vi "UpdateSqueezeRelease.vi"(6 "valley":bool, 7 "valley 2":bool, 9 "peak":bool, 10 "peak 2":bool, 11 "Loop Data":T1) -> (3 "DataLoop":T1)   [LabVIEW 2016]
doc: "updates the number of squeezes nad releases since start of session"
uses:
  DataLoopCluster.ctl
  SignalType.ctl
  range_cluster.ctl
  <userlib>/_OpenG.lib/array/array.llb/Filter 1D Array with Scalar (String)__ogtk.vi
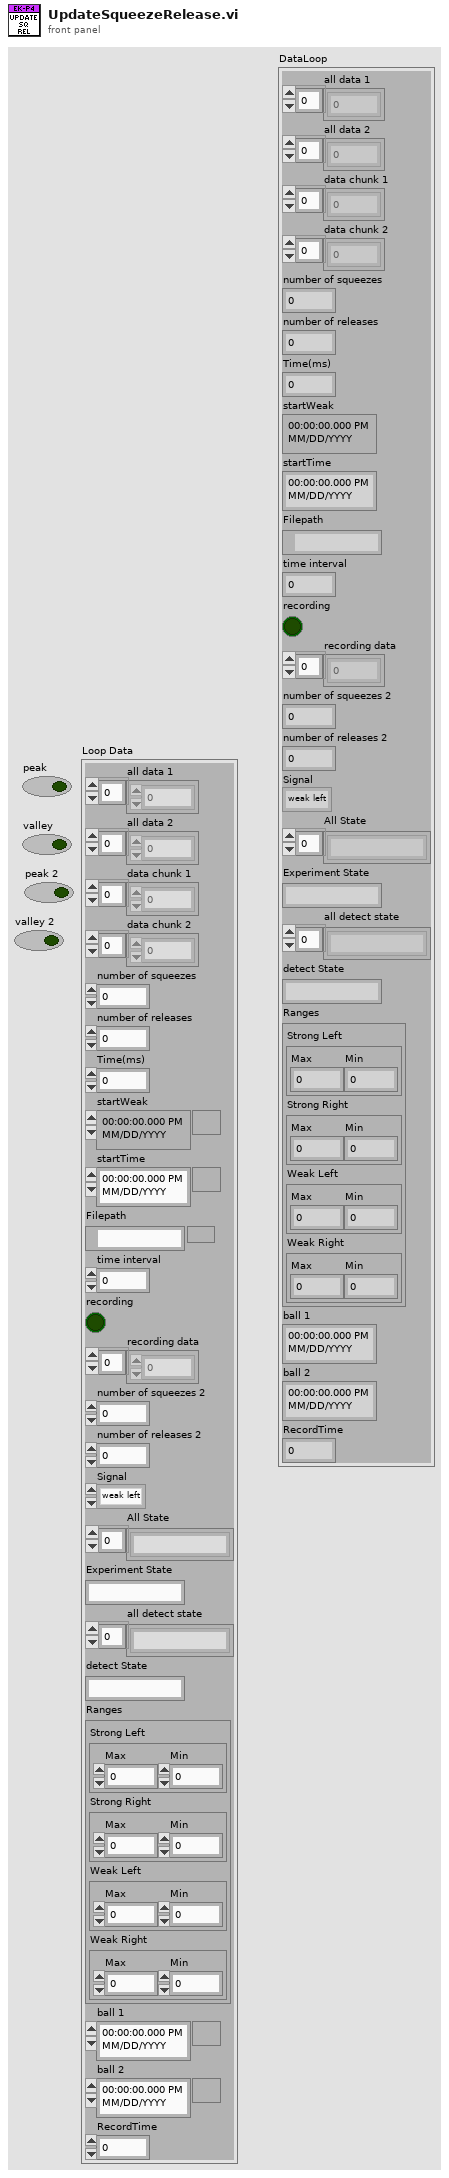
[diagram p1: front panel]
types:
  T1 = typedef "DataLoopCluster.ctl" = cluster{"all data 1":dbl[], "all data 2":dbl[], "data chunk 1":dbl[], "data chunk 2":dbl[], "number of squeezes":u16, "number of releases":u16, "Time(ms)":i64, "startWeak":timestamp, "startTime":timestamp, "Filepath":path, "time interval":u16, "recording":bool, "recording data":dbl[], "number of squeezes 2":u16, "number of releases 2":u16, "Signal":T2, "All State":string[], "Experiment State":string, "all detect state":string[], "detect State":string, "Ranges":cluster{"Strong Left":T3, "Strong Right":T3, "Weak Left":T3, "Weak Right":T3}, "ball 1":timestamp, "ball 2":timestamp, "RecordTime":u16}
  T2 = typedef "SignalType.ctl" = enum16{"weak left", "weak right", "strong left", "strong right"}
  T3 = typedef "range_cluster.ctl" = cluster{"Max":dbl, "Min":dbl}
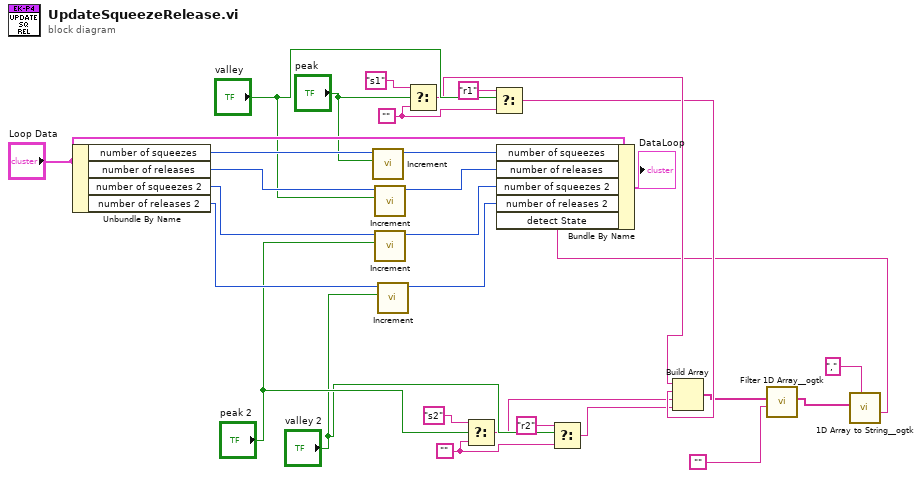
[diagram p0: block diagram]
diagram:
  w13 = ""
  w16 = ""
  n1 = Unbundle By Name("Loop Data") -> ("number of squeezes"=w25:u16, "number of releases"=w29:u16, "number of squeezes 2"=w23:u16, "number of releases 2"=w21:u16)
  n2 = call "Increment.vi"("boolean"="peak", "number in"=w25) -> ("number out"=w24:u16)  [unwired: 9 in]
  n3 = call "Increment.vi"("boolean"="valley", "number in"=w29) -> ("number out"=w27:u16)  [unwired: 9 in]
  n4 = call "Increment.vi"("boolean"="peak 2", "number in"=w23) -> ("number out"=w22:u16)  [unwired: 9 in]
  n5 = call "Increment.vi"("boolean"="valley 2", "number in"=w21) -> ("number out"=w20:u16)  [unwired: 9 in]
  n6 = Select(t="s1", s="peak", f=w16) -> (s? t:f=w9:string)
  n7 = Select(t="s2", s="peak 2", f=w13) -> (s? t:f=w7:string)
  n8 = Select(t="r1", s="valley", f=w16) -> (s? t:f=w8:string)
  n9 = Select(t="r2", s="valley 2", f=w13) -> (s? t:f=w6:string)
  n10 = Build Array(w9, w8, w7, w6) -> (w5:string[])
  n11 = call-poly <userlib>:"Filter 1D Array__ogtk.vi"("items to filter"="", "array"=w5) -> ("filtered array"=w3:string[])  [unwired: 4 in, 1 out]
  n12 = call <userlib>:"1D Array to String__ogtk.vi"("delimiter (Tab)"=",", "Array of Strings"=w3) -> ("delimited string"=w1:string)  [unwired: 9 in]
  n13 = Bundle By Name(cluster="Loop Data", "number of squeezes"=w24, "number of releases"=w27, "number of squeezes 2"=w22, "number of releases 2"=w20, "detect State"=w1) -> (→"DataLoop":T1)
